vi "act-0004-cor.vi"(1 "Deg C":dbl format="%.2f") -> (0 "Deg F":dbl format="%.2f")   [LabVIEW 2010]
doc: "Conversion de degré Celsius en Fahrenheit."
panel:
  # "Ce Vi effectue la conversion de degré Celsius vers degré Fahrenheit"
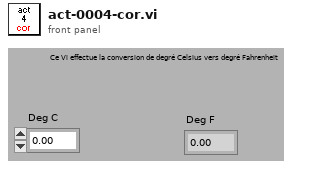
[diagram p1: front panel]
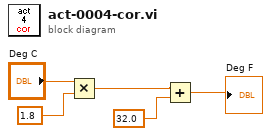
[diagram p0: block diagram]
diagram:
  n1 = Multiply(x="Deg C", y=1.8) -> (x*y=w2:dbl)
  n2 = Add(x=w2, y=32.0) -> (x+y=→"Deg F":dbl)
